vi "SimYokeShin_TP059851_Client.vi"() -> ()   [LabVIEW 2020]
uses:
  <vilib>/Utility/file.llb/Write Delimited Spreadsheet (string).vi
panel:
  out "error out":errorcluster
  in  "App UI":enum32{"Page 1", "Page 2"}(tab)
  in  "Logout Button":bool
  in  "Registration UI":enum32{"Page 1", "Page 2"}(tab)
  in  "Register  Button":bool
  in  "Registration File":string[][](table)
  in  "Login UI":enum32{"Page 1"}(tab)
  out "Status":bool
  in  "Login Button":bool
  in  "Password":string
  in  "User Name":string
  # "Login UI"
  # "Welcome UI"
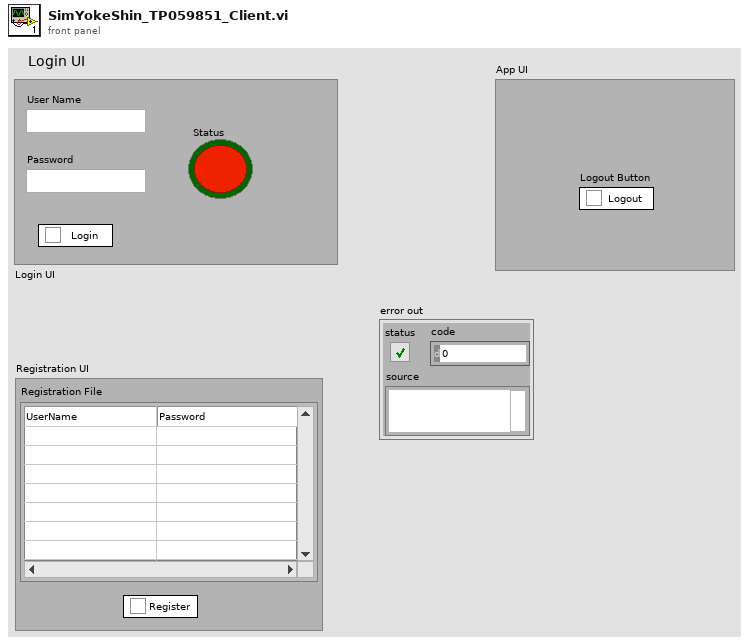
[diagram p1: front panel]
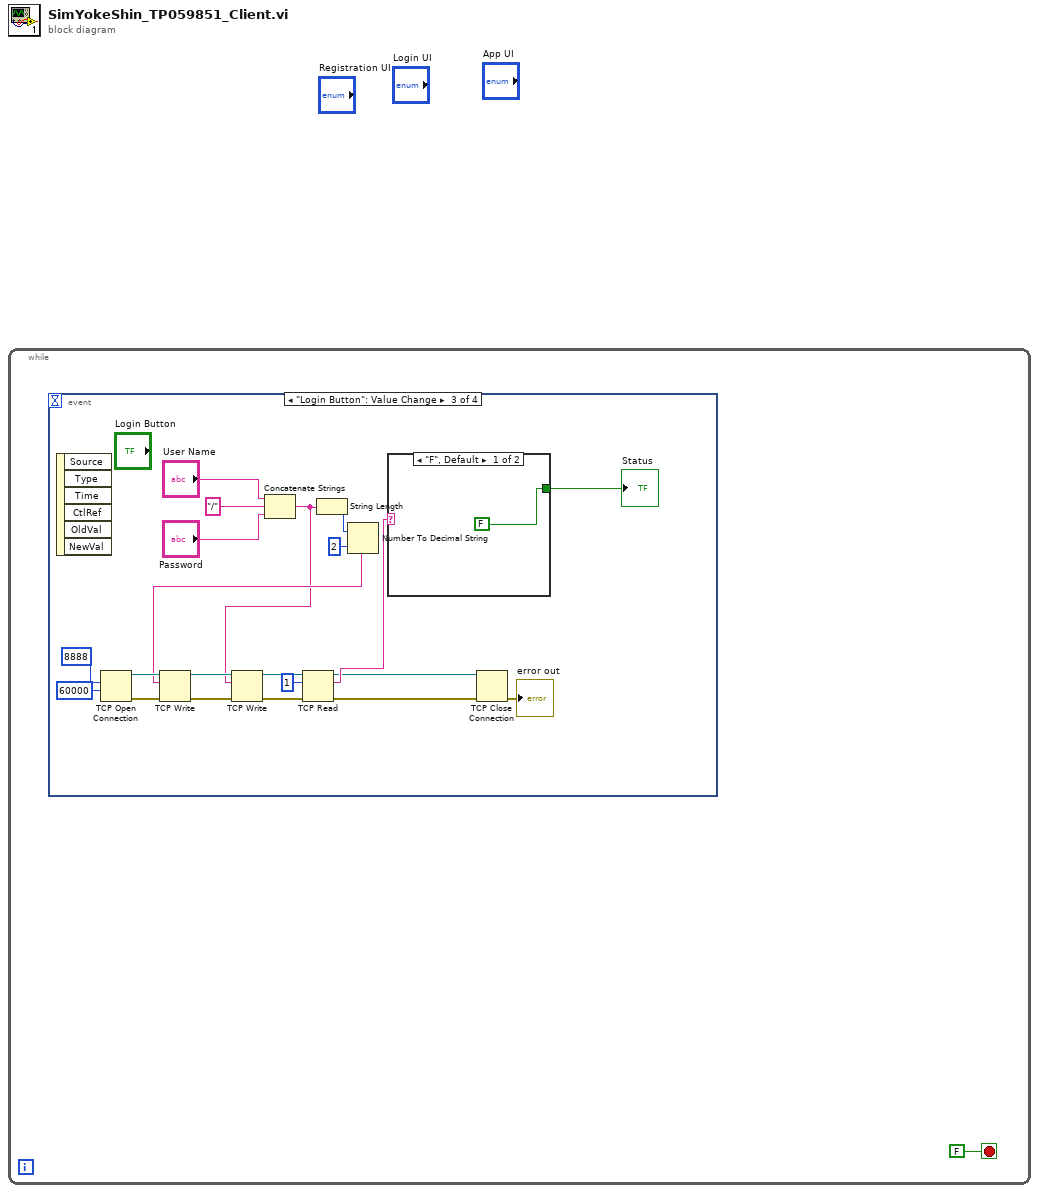
[diagram p0: block diagram]
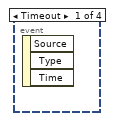
[diagram p2: hidden frame]
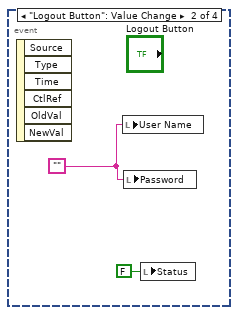
[diagram p3: hidden frame]
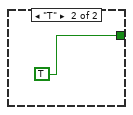
[diagram p4: hidden frame]
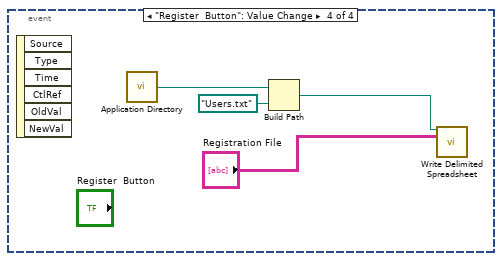
[diagram p5: hidden frame]
diagram:
  n1 = while {
    stop <- FALSE stop-if-true
    n2 = event shown="[2] \"Login Button\": Value Change" {
      selector: _ -> [_ _ _ _]
      dyn-events: _ -> [_ _ _ _]
      timeout: _ -> [_ _ _ _]
      event Timeout {
        n3 = event-data() -> ()  [unwired: 1 in, 3 out]
      }
      event "Logout Button": Value Change {
        w2 = ""
        n4 = event-data() -> ()  [unwired: 1 in, 6 out]
        n5 = local write "User Name"(w2) -> ()
        n6 = local write "Password"(w2) -> ()
        n7 = local write "Status"(FALSE ("Status")) -> ()
      }
      event "Login Button": Value Change {
        n8 = event-data() -> ()  [unwired: 1 in, 6 out]
        n9 = TCP Open Connection(remote port or service name=u16 8888, timeout ms (60000)=60000) -> (connection ID=w19:refnum<k5>, error out=w14:errorcluster)  [unwired: 3 in]
        n10 = Concatenate Strings "Concatenate Strings"("User Name", "/" ("string"), "Password") -> (w10:string)
        n11 = String Length(string=w10) -> (length=w23:i32)
        n12 = Number To Decimal String(number=w23, width (-)=i16 2) -> (decimal integer string=w11:string)
        n13 = TCP Write(connection ID=w19, data in=w11, error in (no error)=w14) -> (connection ID out=w18:refnum<k5>, error out=w15:errorcluster)  [unwired: 1 in, 1 out]
        n14 = TCP Write(connection ID=w18, data in=w10, error in (no error)=w15) -> (connection ID out=w17:refnum<k5>, error out=w16:errorcluster)  [unwired: 1 in, 1 out]
        n15 = TCP Read(connection ID=w17, bytes to read=1, error in (no error)=w16) -> (connection ID out=w5:refnum<k5>, data out=w8:string, error out=w4:errorcluster)  [unwired: 2 in]
        n16 = case shown="\"F\", Default" w8 {
          tunnel: [FALSE TRUE] -> w6
          frame "F", Default {
          }
          frame "T" {
          }
        }
        "Status" <- w6
        n17 = TCP Close Connection(connection ID=w5, error in (no error)=w4) -> (error out=→"error out":errorcluster)  [unwired: 1 in, 1 out]
      }
      event "Register  Button": Value Change {
        n18 = event-data() -> ()  [unwired: 1 in, 6 out]
        n19 = call <vilib>:"Application Directory.vi"() -> ("Application Directory"=w28:path)
        n20 = Build Path(base path=w28, name or relative path=path "Users.txt") -> (appended path=w27:path)
        n21 = call-poly <vilib>:"Write Delimited Spreadsheet.vi"("file path (dialog if empty)"=w27, "2D data"="Registration File") -> ()  [unwired: 12 in, 2 out]
      }
    }
  }
